vi "DCIR_IMAGE.vi"(11 "Bouton Stop":bool) -> ()   [LabVIEW 2020]
uses:
  <userlib>/Alex.vi/FGV.ctl
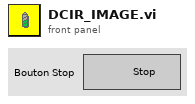
[diagram p1: front panel]
types:
  T1 = typedef "FGV.ctl" = enum16{"GET", "SET", "RAZ"}
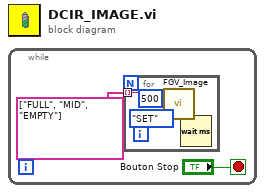
[diagram p0: block diagram]
diagram:
  n1 = while {
    stop <- "Bouton Stop" stop-if-true
    n2 = for {
      tunnel: string[] ["FULL", "MID", "EMPTY"] -> [w4] mode=indexing
      n3 = call <userlib>:"FGV_Image.vi"("Énum"=FGV."SET", "IN"=w4) -> ()  [unwired: 9 in, 1 out]
      n4 = Wait (ms)(milliseconds to wait=u32 500 ("attente (ms)")) -> ()  [unwired: 1 out]
    }
  }
